vi "Proceso Moneda.vi"(8 "error in (no error)":errorcluster, 10 "Coins":cluster{"$1":bool, "$2":bool, "$5":bool}, 11 "USD ACTOR in":refnum<class "USD ACTOR.lvclass">) -> (0 "error out":errorcluster, 3 "USD ACTOR out":refnum<class "USD ACTOR.lvclass">)   [LabVIEW 2019, in "USD ACTOR.lvlib" / "USD ACTOR.lvclass"]
uses:
  USD ACTOR.lvclass
  C:/Program Files (x86)/National Instruments/LabVIEW 2019/vi.lib/ActorFramework/Actor/Actor.lvclass
  <vilib>/ActorFramework/Actor/Actor.lvclass/Actor.ctl
  USD ACTOR.lvclass/USD ACTOR.ctl
  UI Actor Messages/Credit update1 Msg/Credit update1 Msg.lvclass/Credit update1 Msg.ctl
  <vilib>/ActorFramework/Message Enqueuer/Message Enqueuer.lvclass/Message Enqueuer.ctl
  <vilib>/ActorFramework/Message Enqueuer/Enqueue.vi
  UI Actor Messages/Credit update1 Msg/Credit update1 Msg.lvclass
  C:/Program Files (x86)/National Instruments/LabVIEW 2019/vi.lib/ActorFramework/Message/Message.lvclass
  <vilib>/ActorFramework/Message Priority Queue/Priority Enqueue.vi
  <vilib>/ActorFramework/Actor/Actor.lvclass
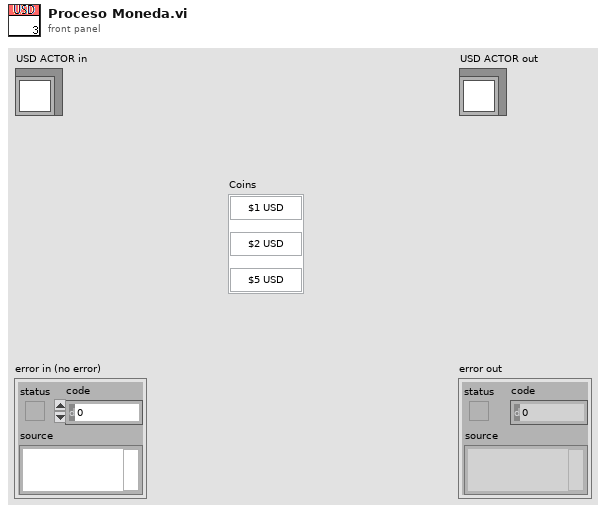
[diagram p1: front panel]
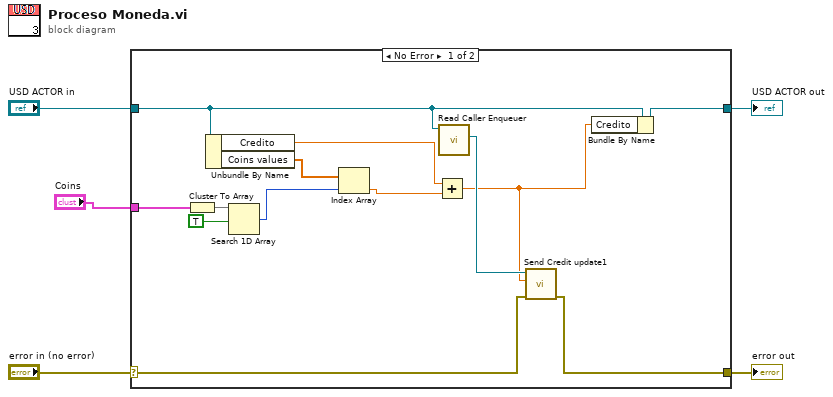
[diagram p0: block diagram]
diagram:
  n1 = case shown="No Error" "error in (no error)" {
    selector: "error in (no error)" -> [w7 w20]
    tunnel: [w6 w20] -> w4
    tunnel: [w12 w19] -> w2
    tunnel: "USD ACTOR in" -> [w13 w19]
    tunnel: "Coins" -> [w18 _]
    frame No Error {
      n2 = Cluster To Array(cluster=w18) -> (array=w17:bool[])
      n3 = Unbundle By Name(w13) -> ("Credito"=w11:dbl, "Coins values"=w14:dbl[])
      n4 = Search 1D Array(1D array=w17, element=TRUE) -> (index of element=w15:i32)  [unwired: 1 in]
      n5 = Index Array(array=w14, index=w15) -> (element=w8:dbl)
      n6 = Add(x=w11, y=w8) -> (x+y=w9:dbl)
      n7 = call <vilib>:"Read Caller Enqueuer.vi"("Actor"=w13) -> ("Caller Enqueuer"=w10:refnum<class "Message Enqueuer.lvclass">)  [unwired: 10 in]
      n8 = call "Send Credit update1.vi"("error in (no error)"=w7, "Credit"=w9, "Message Enqueuer"=w10) -> ("error out"=w6:errorcluster)  [unwired: 7 in, 1 out]
      n9 = Bundle By Name(cluster=w13, "Credito"=w9) -> (w12:refnum<class "USD ACTOR.lvclass">)
    }
    frame Error {
    }
  }
  "error out" <- w4
  "USD ACTOR out" <- w2
